vi "GetCollisionEvents.vi"(11 "Tab Array":string[][](array[string])) -> (3 "Collision Events":cluster{"Depth":dbl[], "D1":dbl[]})   [LabVIEW 2012]
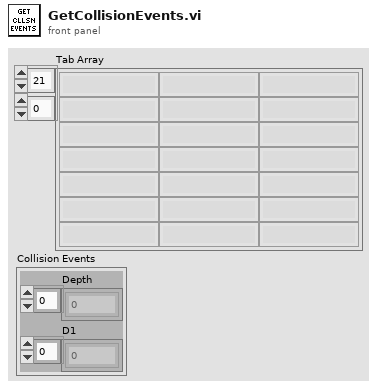
[diagram p1: front panel]
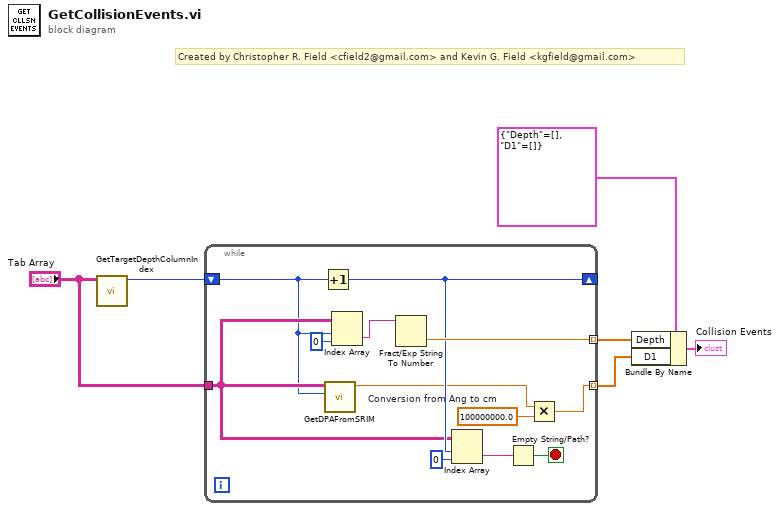
[diagram p0: block diagram]
diagram:
  # "Created by Christopher R. Field <cfield2@gmail.com> and Kevin G. Field <kgfield@gmail.com>"
  n1 = call "GetTargetDepthColumnIndex.vi"("Tab Array"="Tab Array") -> ("Start Index"=w1:i32)  [unwired: 9 in, 1 out]
  n2 = while {
    shift-right: [w14] -> _
    shift-left: w1 -> [w8]
    tunnel: "Tab Array" -> [w9]
    tunnel: [w10] -> w4 mode=indexing
    tunnel: [w16] -> w5 mode=indexing
    stop <- w12 stop-if-true
    w11 = 100000000.0  # Conversion from Ang to cm
    n3 = Increment(x=w8) -> (x+1=w14:i32)
    n4 = call "GetDPAFromSRIM.vi"("Start Index"=w8, "Tab Array"=w9) -> ("DPA"=w7:dbl)  [unwired: 9 in]
    n5 = Index Array(array=w9, index (row)=w8, index (col)=0 ("disabled index (col)")) -> (element=w18:string)
    n6 = Fract/Exp String To Number(string=w18) -> (number=w16:dbl)  [unwired: 3 in, 1 out]
    n7 = Index Array(array=w9, index (row)=w14, index (col)=0 ("disabled index (col)")) -> (element=w13:string)
    n8 = Empty String/Path?(string/path=w13) -> (empty?=w12:bool)
    n9 = Multiply(x=w7, y=w11) -> (x*y=w10:dbl)
  }
  n10 = Bundle By Name(cluster=cluster{"Depth":dbl[], "D1":dbl[]} {"Depth"=[], "D1"=[]}, "Depth"=w5, "D1"=w4) -> (→"Collision Events":cluster{"Depth":dbl[], "D1":dbl[]})
